vi "Write A_msg Msg.vi"(10 "A_Actor.lvlib:A_msg Msg.lvclass":refnum<class "A_msg Msg.lvclass">, 11 "A_Actor in":refnum<class "A_Actor.lvclass">) -> (3 "A_Actor out":refnum<class "A_Actor.lvclass">)   [LabVIEW 2025, in "A_Actor.lvlib" / "A_Actor.lvclass"]
uses:
  A_Actor.lvclass
  A_Actor Messages/A_msg Msg/A_msg Msg.lvclass
  A_Actor.lvclass/A_Actor.ctl
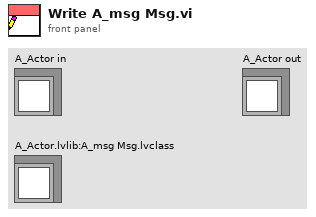
[diagram p1: front panel]
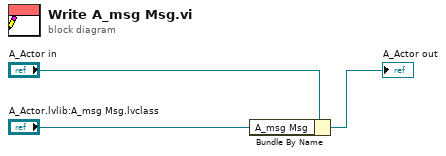
[diagram p0: block diagram]
diagram:
  n1 = Bundle By Name(cluster="A_Actor in", "A_msg Msg"="A_Actor.lvlib:A_msg Msg.lvclass") -> (→"A_Actor out":refnum<class "A_Actor.lvclass">)
